vi "Get CD Storage Library Loader Ref.vi"(11 "DMA Channel Testing in":refnum<class "DMA Channel Testing.lvclass">) -> (2 "CDS Loader Ref":refnum<vi>, 3 "DMA Channel Testing out":refnum<class "DMA Channel Testing.lvclass">)   [LabVIEW 2019, in "DMA Channel Testing.lvclass"]
uses:
  DMA Channel Testing.lvclass
  DMA Channel Testing.lvclass/DMA Channel Testing.ctl
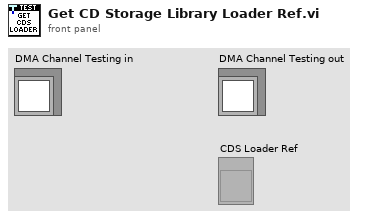
[diagram p1: front panel]
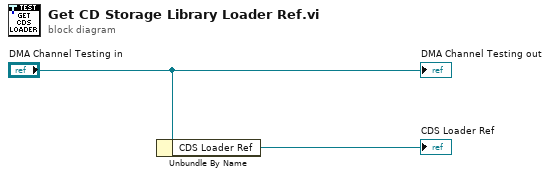
[diagram p0: block diagram]
diagram:
  n1 = Unbundle By Name("DMA Channel Testing in") -> ("CDS Loader Ref"=→"CDS Loader Ref":refnum<vi>)
  "DMA Channel Testing out" <- "DMA Channel Testing in"
